vi "App_Update Data.vi"(8 "error in":errorcluster, 11 "Live Mode?(F)":bool) -> (0 "error out":errorcluster, 3 "Data":waveform(dbl), 5 "Update Result":T1)   [LabVIEW 2015, in "Application 1.lvlib"]
uses:
  Application 1.lvlib
  Com VIs/Data Def/Update Result.ctl
  Data Def/App_Simulator Data Method.ctl
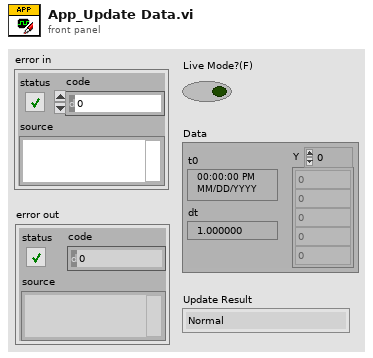
[diagram p1: front panel]
types:
  T1 = typedef "Update Result.ctl" = enum16{"Normal", "Abnormal", "Can't find training data"}
  T2 = typedef "Application 1.lvlib/App_Simulator Data Method.ctl" = enum16{"Get", "Put"}
  T3 = typedef "Application 1.lvlib/App_Main Data.ctl" = cluster{"VI Refnum":refnum<vi>, "Subpanel":refnum<vi>, "Connection ID":refnum<k5>, "Meta data":T4[], "Main Queue":T6, "User Data":T7}
  T4 = typedef "stm_MetaElement.ctl" = cluster{"Name":T5}
  T5 = typedef "stm_MetaDataElement.ctl" = string
  T6 = typedef "Application 1.lvlib/App_Main Queue.ctl" = cluster{"Main Loop Queue":refnum<queue>}
  T7 = typedef "User Data.ctl" = cluster{"Name":string, "Email":string, "Phone Number":string, "User Picture":u32[][], "Last Login Time":timestamp}
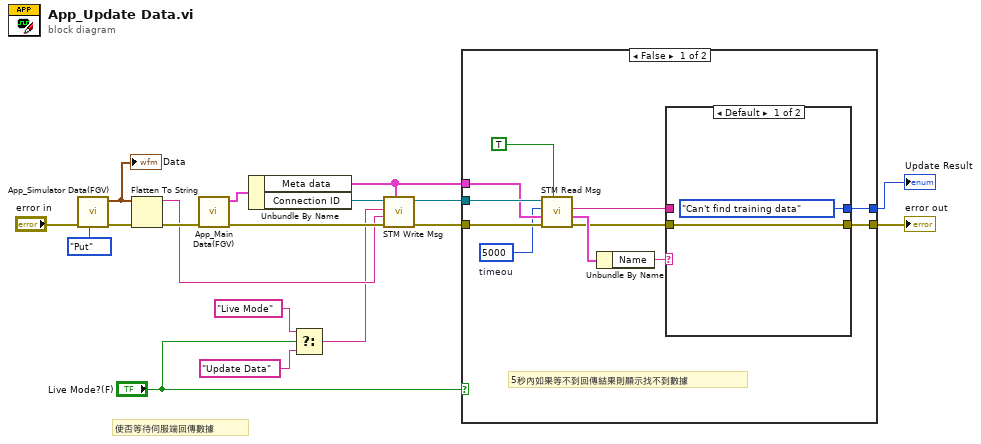
[diagram p0: block diagram]
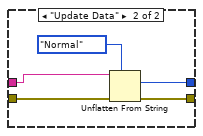
[diagram p2: hidden frame]
diagram:
  # "使否等待伺服端回傳數據"
  n1 = call "App_Simulator Data(FGV).vi"("Simulator Data Method(Get)"=App_Simulator_Data_Method."Put", "error in"="error in") -> ("error out"=w14:errorcluster, "Data"=w11:waveform(dbl))  [unwired: 8 in]
  "Data" <- w11
  n2 = Flatten To String(anything=w11, error in (no error)=w14) -> (data string=w12:string, error out=w13:errorcluster)  [unwired: 2 in, 1 out]
  n3 = call "App_Main Data(FGV).vi"("error in"=w13) -> ("error out"=w16:errorcluster, "Main Data Out"=w17:T3)  [unwired: 9 in]
  n4 = Unbundle By Name(w17) -> ("Meta data"=w4:T4[], "Connection ID"=w15:refnum<k5>)
  n5 = Select(t="Live Mode" ("Name"), s="Live Mode?(F)", f="Update Data" ("Name")) -> (s? t:f=w7:string)
  n6 = call "STM Write Msg.vi"("Meta data"=w4, "error in (no error)"=w16, "Data"=w12, "Name"=w7, "connection ID"=w15) -> ("error out"=w6:errorcluster, "connection ID out"=w5:refnum<k5>)  [unwired: 5 in]
  n7 = case shown="False" "Live Mode?(F)" {
    tunnel: w6 -> [w29 w37]
    tunnel: w5 -> [w28 _]
    tunnel: w4 -> [w27 _]
    tunnel: [w20 _] -> w1
    tunnel: [w19 w37] -> w2
    frame False {
      w26 = 5000  # timeou
      # "5秒內如果等不到回傳結果則顯示找不到數據"
      n8 = call "STM Read Msg.vi"("Ignore Timeout Error"=TRUE, "error in"=w29, "Meta data"=w27, "timeout ms (25000)"=w26, "connection ID"=w28) -> ("error out"=w21:errorcluster, "Meta element"=w24:T4, "data string"=w22:string)  [unwired: 1 in, 3 out]
      n9 = Unbundle By Name(w24) -> ("Name"=w23:T5)
      n10 = case shown="Default" w23 {
        tunnel: w22 -> [_ w35]
        tunnel: w21 -> [w31 w36]
        tunnel: [w31 w33] -> w19
        tunnel: [Update_Result."Can't find training data" ("Update Result") w32] -> w20
        frame Default {
        }
        frame "Update Data" {
          n11 = Unflatten From String(type=Update_Result."Normal" ("Update Result"), binary string=w35, error in (no error)=w36) -> (value=w32:T1, error out=w33:errorcluster)  [unwired: 2 in, 1 out]
        }
      }
    }
    frame True {
    }
  }
  "error out" <- w2
  "Update Result" <- w1
